vi "Sandbox.vi"() -> ()   [LabVIEW 2017]
panel:
  out "Boolean array":bool[](array[boolean])
  out "Remainder":u64
  in  "SizeBytes":u64=32
  out "Remainder":u64
  out "Quotient":u64
  out "TotalWords":u64
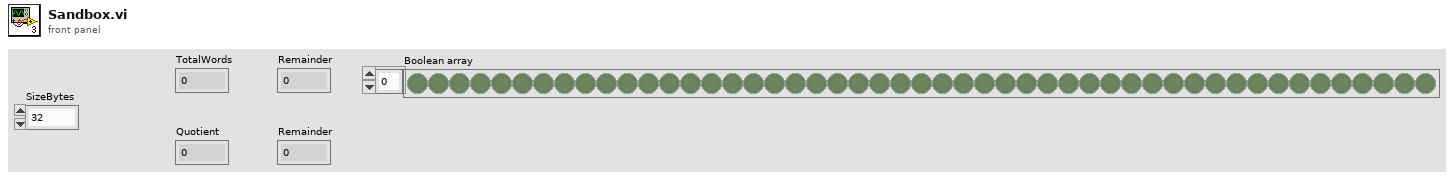
[diagram p1: front panel]
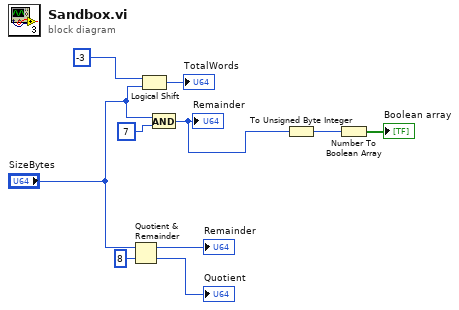
[diagram p0: block diagram]
diagram:
  n1 = Quotient & Remainder(x="SizeBytes", y=u64 8) -> (x-y*floor(x/y)=→"Remainder":u64, floor(x/y)=→"Quotient":u64)
  n2 = Logical Shift(y=i16 -3, x="SizeBytes") -> (x << y=→"TotalWords":u64)
  n3 = And(x="SizeBytes", y=u64 7) -> (x .and. y?=w3:u64)
  "Remainder" <- w3
  n4 = To Unsigned Byte Integer(number=w3) -> (unsigned 8bit integer=w1:u8)
  n5 = Number To Boolean Array(number=w1) -> (Boolean array=→"Boolean array":bool[])
